vi "subvi.vi"(11 "tab liczb R":dbl[](array[numeric])) -> (3 "indeks":i32[](array[numeric]))   [LabVIEW 2013]
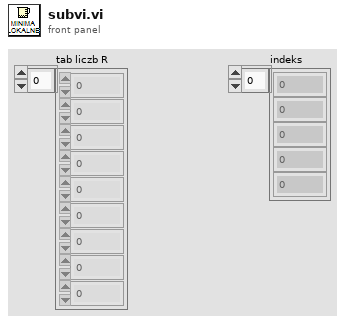
[diagram p1: front panel]
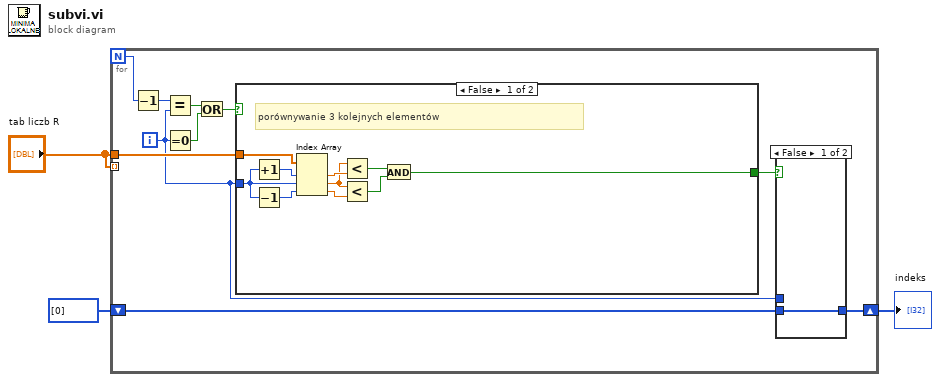
[diagram p0: block diagram]
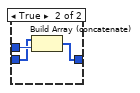
[diagram p2: hidden frame]
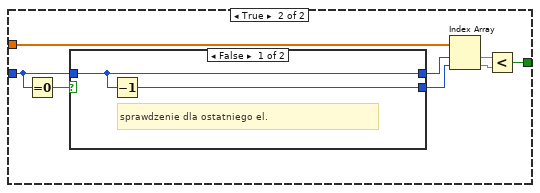
[diagram p3: hidden frame]
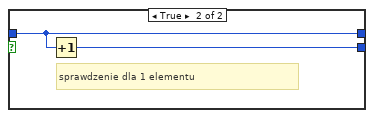
[diagram p4: hidden frame]
diagram:
  n1 = for {
    N -> [w7]
    tunnel: "tab liczb R" -> [_] mode=indexing
    tunnel: "tab liczb R" -> [w8]
    shift-right: [w6] -> w2
    shift-left: i32[] [0] -> [w9]
    i -> [w4]
    n2 = Decrement(x=w7) -> (x-1=w13:i32)
    n3 = Equal?(x=w13, y=w4) -> (x = y?=w12:bool)
    n4 = Equal To 0?(x=w4) -> (x = 0?=w11:bool)
    n5 = Or(x=w12, y=w11) -> (x .or. y?=w10:bool)
    n6 = case shown="False" w10 {
      tunnel: w8 -> [w27 w34]
      tunnel: w4 -> [w19 w30]
      tunnel: [w18 w28] -> w5
      frame False {
        # "porównywanie 3 kolejnych elementów"
        n7 = Increment(x=w19) -> (x+1=w26:i32)
        n8 = Decrement(x=w19) -> (x-1=w25:i32)
        n9 = Index Array(array=w27, index #1=w26, index #2=w19, index #3=w25) -> (element #1=w21:dbl, element #2=w20:dbl, element #3=w24:dbl)
        n10 = Less?(x=w20, y=w21) -> (x < y?=w23:bool)
        n11 = Less?(x=w20, y=w24) -> (x < y?=w22:bool)
        n12 = And(x=w23, y=w22) -> (x .and. y?=w18:bool)
      }
      frame True {
        n13 = Equal To 0?(x=w30) -> (x = 0?=w35:bool)
        n14 = case shown="False" w35 {
          tunnel: w30 -> [w36 w39]
          tunnel: [w36 w39] -> w29
          tunnel: [w37 w38] -> w33
          frame False {
            # "sprawdzenie dla ostatniego el."
            n15 = Decrement(x=w36) -> (x-1=w37:i32)
          }
          frame True {
            # "sprawdzenie dla 1 elementu"
            n16 = Increment(x=w39) -> (x+1=w38:i32)
          }
        }
        n17 = Index Array(array=w34, index #1=w29, index #2=w33) -> (element #1=w31:dbl, element #2=w32:dbl)
        n18 = Less?(x=w31, y=w32) -> (x < y?=w28:bool)
      }
    }
    n19 = case shown="False" w5 {
      tunnel: w9 -> [w14 w15]
      tunnel: w4 -> [_ w17]
      tunnel: [w14 w16] -> w6
      frame False {
      }
      frame True {
        n20 = Build Array (concatenate)(w15, w17) -> (w16:i32[])
      }
    }
  }
  "indeks" <- w2
